vi "CTRE_Phoenix_MotorControl_ConfigGetAllCustomParameters.vi"(6 "timeoutMs":i32=50, 11 "PhoenixMotorControlDevRef in":T1) -> (0 "AnyConfigGetFailed":bool, 2 "CustomParam 2":T6, 3 "PhoenixMotorControlDevRef out":T1)   [LabVIEW 2017]
uses:
  <vilib>/Rock Robotics/WPI/MotorControl/WPI_MotorControlDeviceRef.ctl
  <vilib>/Rock Robotics/WPI/MotorControl/WPI_MotorControlType.ctl
  <vilib>/Rock Robotics/SystemInterfaces/DIO/FPGA_DIOPWMChannel.ctl
  <vilib>/Rock Robotics/WPI/PWM/WPI_PWMDeadband.ctl
  <vilib>/Rock Robotics/SystemInterfaces/DIO/FPGA_DIOChannel.ctl
  <vilib>/Rock Robotics/WPI/ThirdParty/Phoenix-LabVIEW/Controls/CTRE_Phoenix_CustomParamConfiguration.ctl
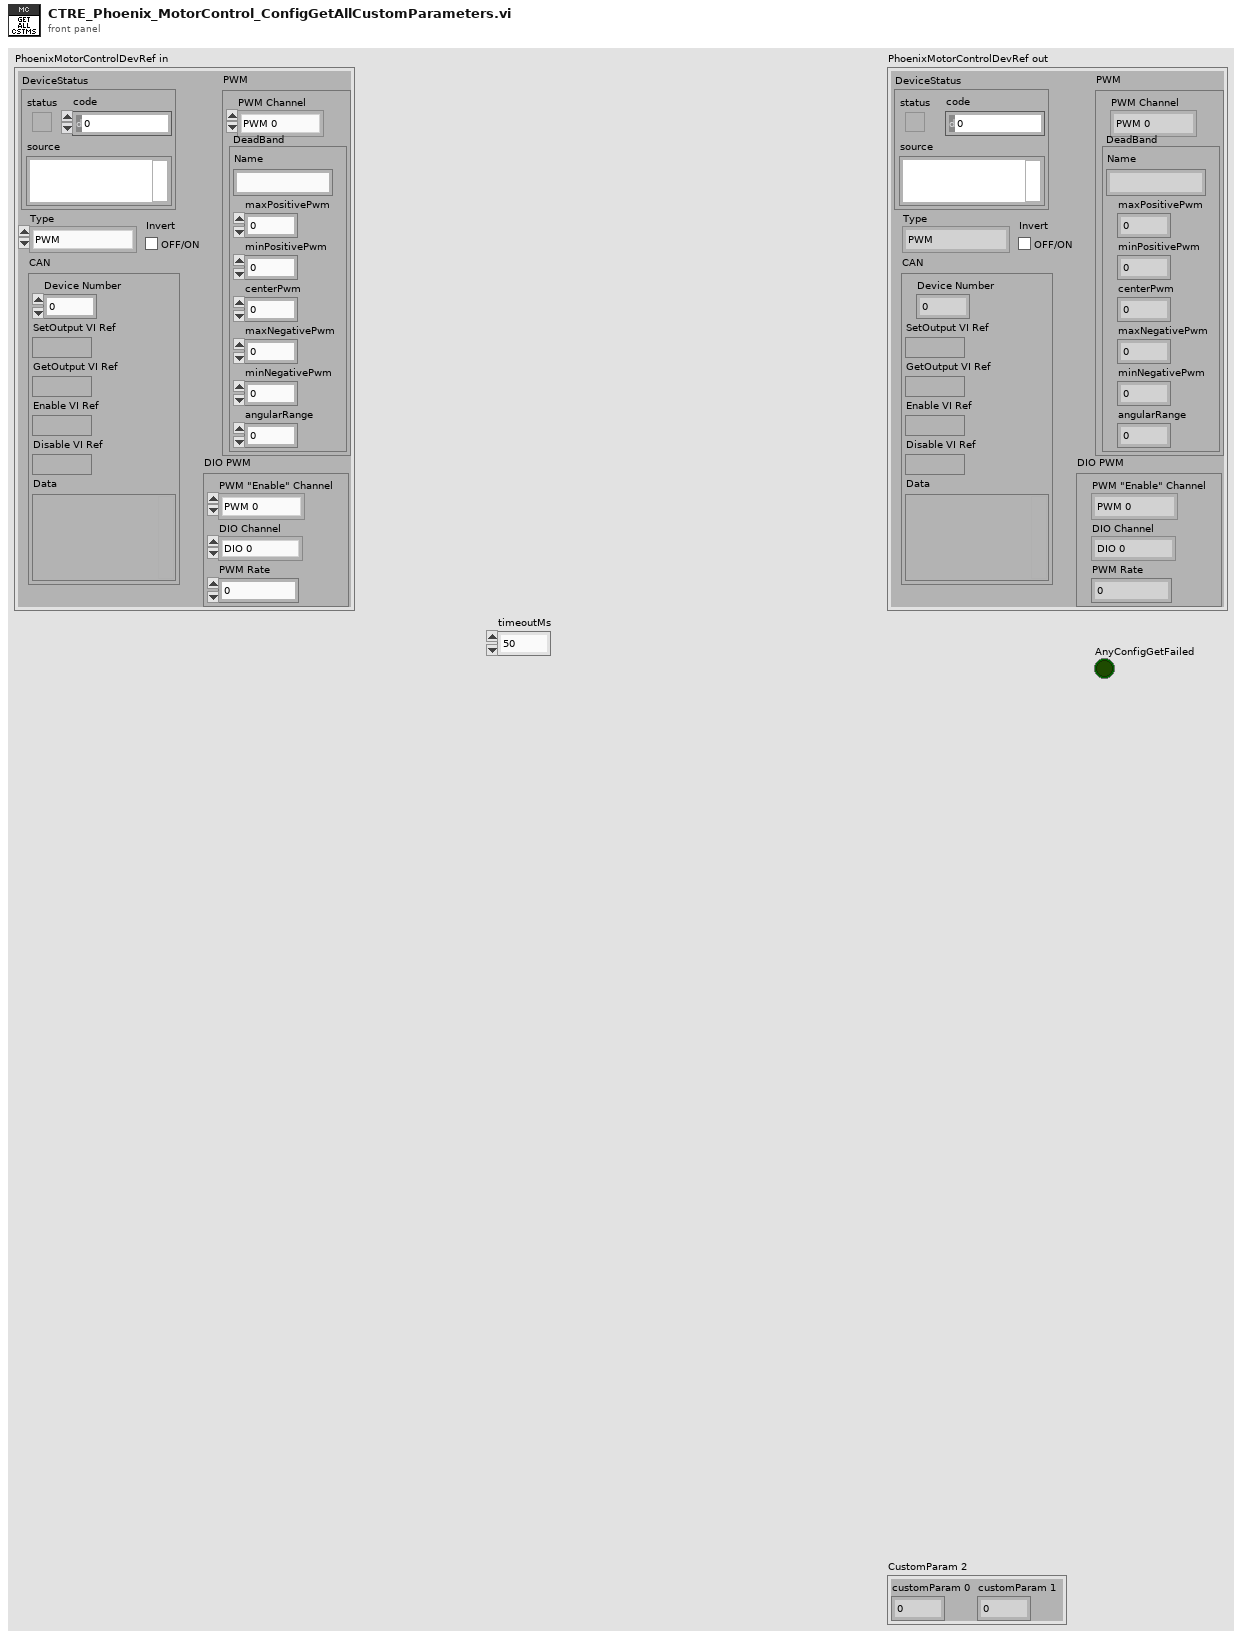
[diagram p1: front panel]
types:
  T1 = typedef "WPI_MotorControlDeviceRef.ctl" = cluster{"DeviceStatus":errorcluster, "Type":T2, "PWM":cluster{"PWM Channel":T3, "DeadBand":T4}, "CAN":cluster{"Device Number":u8, "SetOutput VI Ref":variant, "GetOutput VI Ref":variant, "Enable VI Ref":variant, "Disable VI Ref":variant, "Data":variant}, "Invert":bool, "DIO PWM":cluster{"PWM \"Enable\" Channel":T3, "DIOChannel":T5, "PWM Rate":dbl}}
  T2 = typedef "WPI_MotorControlType.ctl" = enum16{"PWM", "CAN", "DIO PWM"}
  T3 = typedef "FPGA_DIOPWMChannel.ctl" = enum8{"PWM 0", "PWM 1", "PWM 2", "PWM 3", "PWM 4", "PWM 5", "PWM 6", "PWM 7", "PWM 8", "PWM 9", "PWM MXP 0", "PWM MXP 1", "PWM MXP 2", "PWM MXP 3", "PWM MXP 4", "PWM MXP 5", "PWM MXP 6", "PWM MXP 7", "PWM MXP 8", "PWM MXP 9", "Invalid"}
  T4 = typedef "WPI_PWMDeadband.ctl" = cluster{"Name":string, "maxPositivePwm":i32, "minPositivePwm":i32, "centerPwm":i32, "maxNegativePwm":i32, "minNegativePwm":i32, "angularRange":u16}
  T5 = typedef "FPGA_DIOChannel.ctl" = enum8{"DIO 0", "DIO 1", "DIO 2", "DIO 3", "DIO 4", "DIO 5", "DIO 6", "DIO 7", "DIO 8", "DIO 9", "DIO MXP 0", "DIO MXP 1", "DIO MXP 2", "DIO MXP 3", "DIO MXP 4", "DIO MXP 5", "DIO MXP 6", "DIO MXP 7", "DIO MXP 8", "DIO MXP 9", "DIO MXP 10", "DIO MXP 11", "DIO MXP 12", "DIO MXP 13", "DIO MXP 14", "DIO MXP 15", "SPI Port CS1", "SPI Port CS2", "SPI Port CS3", "SPI Port MISO", "SPI Port MOSI", "Invalid"}
  T6 = typedef "CTRE_Phoenix_CustomParamConfiguration.ctl" = cluster{"customParam 0":i32, "customParam 1":i32}
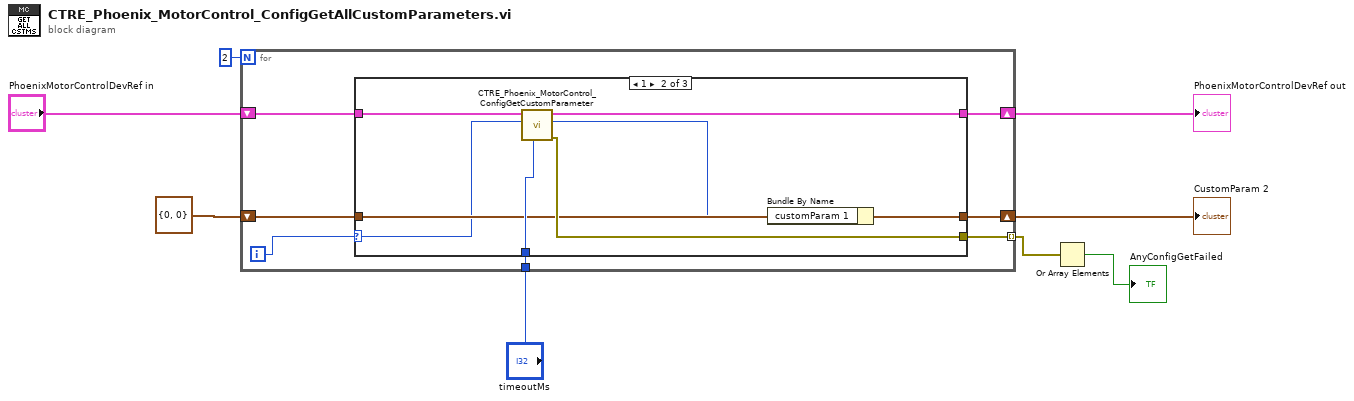
[diagram p0: block diagram]
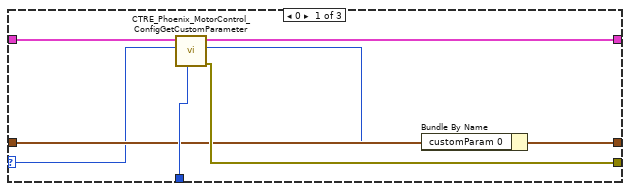
[diagram p2: hidden frame]
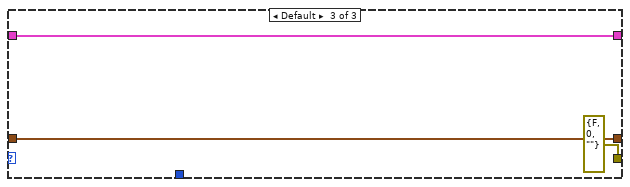
[diagram p3: hidden frame]
diagram:
  n1 = for {
    N: 2 -> [_]
    tunnel: [w13] -> w3 mode=indexing
    tunnel: "timeoutMs" -> [w12]
    shift-right: [w14] -> w7
    shift-left: T6 {"customParam 0"=0, "customParam 1"=0} ("CustomParam") -> [w11]
    shift-right: [w15] -> w8
    shift-left: "PhoenixMotorControlDevRef in" -> [w10]
    i -> [w9]
    n2 = case shown="1" w9 {
      selector: w9 -> [w16 w24 _]
      tunnel: [w23 w31 w34] -> w15
      tunnel: [w22 w30 w33] -> w14
      tunnel: [w21 w29 errorcluster {"status"=FALSE, "code"=0, "source"=""} ("error out")] -> w13
      tunnel: w12 -> [w20 w28 _]
      tunnel: w11 -> [w19 w27 w33]
      tunnel: w10 -> [w18 w26 w34]
      frame 0 {
        n3 = call <vilib>:"CTRE_Phoenix_MotorControl_ConfigGetCustomParameter.vi"("timeoutMs"=w20, "paramIdx"=w16, "PhoenixMotorControlDevRef"=w18) -> ("error out"=w21:errorcluster, "readValue"=w17:i32, "PhoenixMotorControlDevRef"=w23:T1)  [unwired: 6 in]
        n4 = Bundle By Name(cluster=w19, "customParam 0"=w17) -> (w22:T6)
      }
      frame 1 {
        n5 = call <vilib>:"CTRE_Phoenix_MotorControl_ConfigGetCustomParameter.vi"("timeoutMs"=w28, "paramIdx"=w24, "PhoenixMotorControlDevRef"=w26) -> ("error out"=w29:errorcluster, "readValue"=w25:i32, "PhoenixMotorControlDevRef"=w31:T1)  [unwired: 6 in]
        n6 = Bundle By Name(cluster=w27, "customParam 1"=w25) -> (w30:T6)
      }
      frame Default {
      }
    }
  }
  "PhoenixMotorControlDevRef out" <- w8
  "CustomParam 2" <- w7
  n7 = Or Array Elements(Boolean array=w3) -> (logical OR=→"AnyConfigGetFailed":bool)
